vi "detect_bool_changes.vi"(5 "Time has Elapsed 5":bool, 6 "Cluster in":T1, 7 "Time has Elapsed 4":bool, 9 "Time has Elapsed":bool, 10 "Time has Elapsed 2":bool, 11 "Time has Elapsed 3":bool) -> (1 "String":string, 3 "Boolean out":bool)   [LabVIEW 2017]
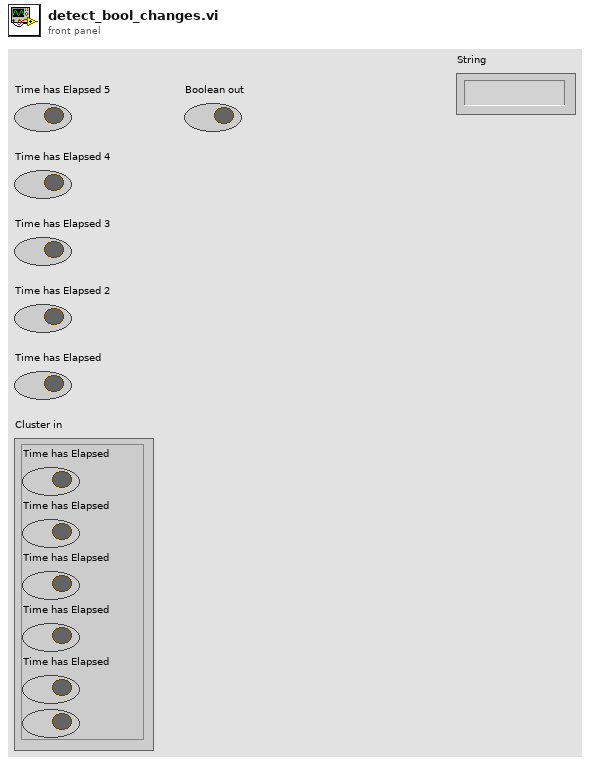
[diagram p1: front panel]
types:
  T1 = cluster{"Time has Elapsed":bool, "Time has Elapsed":bool, "Time has Elapsed":bool, "Time has Elapsed":bool, "Time has Elapsed":bool, "Boolean":bool}
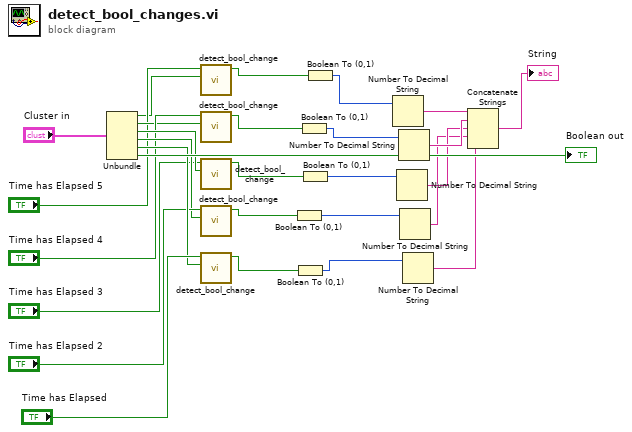
[diagram p0: block diagram]
diagram:
  n1 = Unbundle("Cluster in") -> ("Time has Elapsed"=w18:bool, "Time has Elapsed"=w20:bool, "Time has Elapsed"=w23:bool, "Time has Elapsed"=w24:bool, "Time has Elapsed"=w26:bool, "Boolean"=→"Boolean out":bool)
  n2 = call "detect_bool_change.vi"("Boolean in"=w18, "Boolean 3"="Time has Elapsed 5") -> ("Boolean out"=w16:bool)  [unwired: 9 in]
  n3 = call "detect_bool_change.vi"("Boolean in"=w20, "Boolean 3"="Time has Elapsed 4") -> ("Boolean out"=w15:bool)  [unwired: 9 in]
  n4 = call "detect_bool_change.vi"("Boolean in"=w23, "Boolean 3"="Time has Elapsed 3") -> ("Boolean out"=w14:bool)  [unwired: 9 in]
  n5 = call "detect_bool_change.vi"("Boolean in"=w24, "Boolean 3"="Time has Elapsed 2") -> ("Boolean out"=w13:bool)  [unwired: 9 in]
  n6 = call "detect_bool_change.vi"("Boolean in"=w26, "Boolean 3"="Time has Elapsed") -> ("Boolean out"=w12:bool)  [unwired: 9 in]
  n7 = Boolean To (0,1)(Boolean=w13) -> (0, 1=w8:i16)
  n8 = Boolean To (0,1)(Boolean=w12) -> (0, 1=w7:i16)
  n9 = Boolean To (0,1)(Boolean=w15) -> (0, 1=w10:i16)
  n10 = Boolean To (0,1)(Boolean=w14) -> (0, 1=w9:i16)
  n11 = Boolean To (0,1)(Boolean=w16) -> (0, 1=w11:i16)
  n12 = Number To Decimal String(number=w11) -> (decimal integer string=w6:string)  [unwired: 1 in]
  n13 = Number To Decimal String(number=w9) -> (decimal integer string=w4:string)  [unwired: 1 in]
  n14 = Number To Decimal String(number=w10) -> (decimal integer string=w5:string)  [unwired: 1 in]
  n15 = Number To Decimal String(number=w8) -> (decimal integer string=w3:string)  [unwired: 1 in]
  n16 = Number To Decimal String(number=w7) -> (decimal integer string=w2:string)  [unwired: 1 in]
  n17 = Concatenate Strings(w6, w5, w4, w3, w2) -> (→"String":string)
